vi "Get SMO HELP.vi"(8 "error in (no error)":errorcluster, 10 "Command":string, 11 "Inst.Krohn-Hite-7008 in":refnum<class "Inst.Krohn-Hite-7008.lvclass">) -> (0 "error out":errorcluster, 2 "help cluster":T1, 3 "Inst.Krohn-Hite-7008 out":refnum<class "Inst.Krohn-Hite-7008.lvclass">)   [LabVIEW 2019, in "Inst.Krohn-Hite-7008.lvclass"]
uses:
  Inst.Krohn-Hite-7008.lvclass
  <userlib>/LevyLab/Instrument Framework/subsystems/Help/typedefs/Help--cluster.ctl
  Typedefs/getChannelRequest--Cluster.ctl
  KH7008/typedefs/channel--numeric.ctl
  Typedefs/getAllChannelsResponse--Cluster.ctl
  KH7008/typedefs/allChannelProperties--Array.ctl
  KH7008/typedefs/channelProperties--Cluster.ctl
  KH7008/typedefs/gain--enum.ctl
  KH7008/typedefs/Input--Enum.ctl
  KH7008/typedefs/shunt--enum.ctl
  KH7008/typedefs/couple--Enum.ctl
  KH7008/typedefs/Filter--Enum.ctl
  Typedefs/setChannelRequest--Cluster.ctl
  Typedefs/setAllChannelsRequest--Cluster.ctl
  <userlib>/LevyLab/Instrument Framework/Instrument Types/Amplifier/Instrument.Amplifier.lvclass
  <userlib>/LevyLab/Instrument Framework/subsystems/Help/Help.lvclass
  <userlib>/LevyLab/Instrument Framework/Instrument/Typedefs/Instrument.Commands--Enum.ctl
  <vilib>/PRIrvin/JSON-Schema/JSON-Schema.lvlib
  KH7008/KH7008.lvlib
  <userlib>/LevyLab/Instrument Framework/Instrument/Typedefs/Instrument.IDN--cluster.ctl
  <userlib>/LevyLab/Instrument Framework/Instrument/Instrument.lvclass
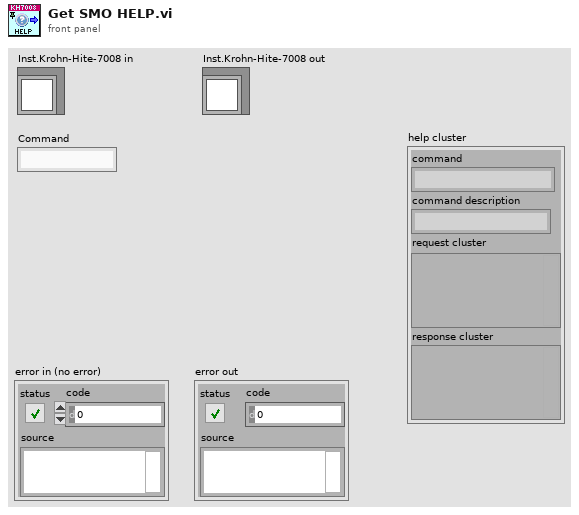
[diagram p1: front panel]
types:
  T1 = typedef "Instrument.lvlib/Help.lvclass/Help--cluster.ctl" = cluster{"command":string, "command description":string, "request cluster":variant, "response cluster":variant}
  T2 = typedef "Inst.Krohn-Hite-7008.lvclass/getAllChannelsResponse--Cluster.ctl" = cluster{"allChannelProperties":T3}
  T3 = typedef "KH7008.lvlib/allChannelProperties--Array.ctl" = T4[]
  T4 = typedef "KH7008.lvlib/channelProperties--Cluster.ctl" = cluster{"channel":T5, "gain":T6, "input":T7, "shunt":T8, "couple":T9, "filter":T10}
  T5 = typedef "KH7008.lvlib/channel--numeric.ctl" = u16
  T6 = typedef "KH7008.lvlib/gain--enum.ctl" = enum16{"1", "10", "100", "1000"}
  T7 = typedef "KH7008.lvlib/Input--Enum.ctl" = enum16{"OFF", "SE+", "SE-", "DIFF"}
  T8 = typedef "KH7008.lvlib/shunt--enum.ctl" = enum16{"Open", "50", "500", "5k", "50k", "10M"}
  T9 = typedef "KH7008.lvlib/couple--Enum.ctl" = enum16{"AC", "DC"}
  T10 = typedef "KH7008.lvlib/Filter--Enum.ctl" = enum16{"OFF", "ON"}
  T11 = typedef "Inst.Krohn-Hite-7008.lvclass/getChannelRequest--Cluster.ctl" = cluster{"channel":T5}
  T12 = typedef "Inst.Krohn-Hite-7008.lvclass/setChannelRequest--Cluster.ctl" = cluster{"channelProperties":T4}
  T13 = typedef "Inst.Krohn-Hite-7008.lvclass/setAllChannelsRequest--Cluster.ctl" = cluster{"allChannelProperties":T3}
  T14 = typedef "Instrument.lvclass/Instrument.Commands--Enum.ctl" = enum16{"ACK", "HELP", "IDN", "getAll", "getAllData"}
  T15 = typedef "Instrument.lvlib/Instrument.lvclass/Instrument.IDN--cluster.ctl" = cluster{"vendor":string, "model":string, "serial":string, "firmware":string}
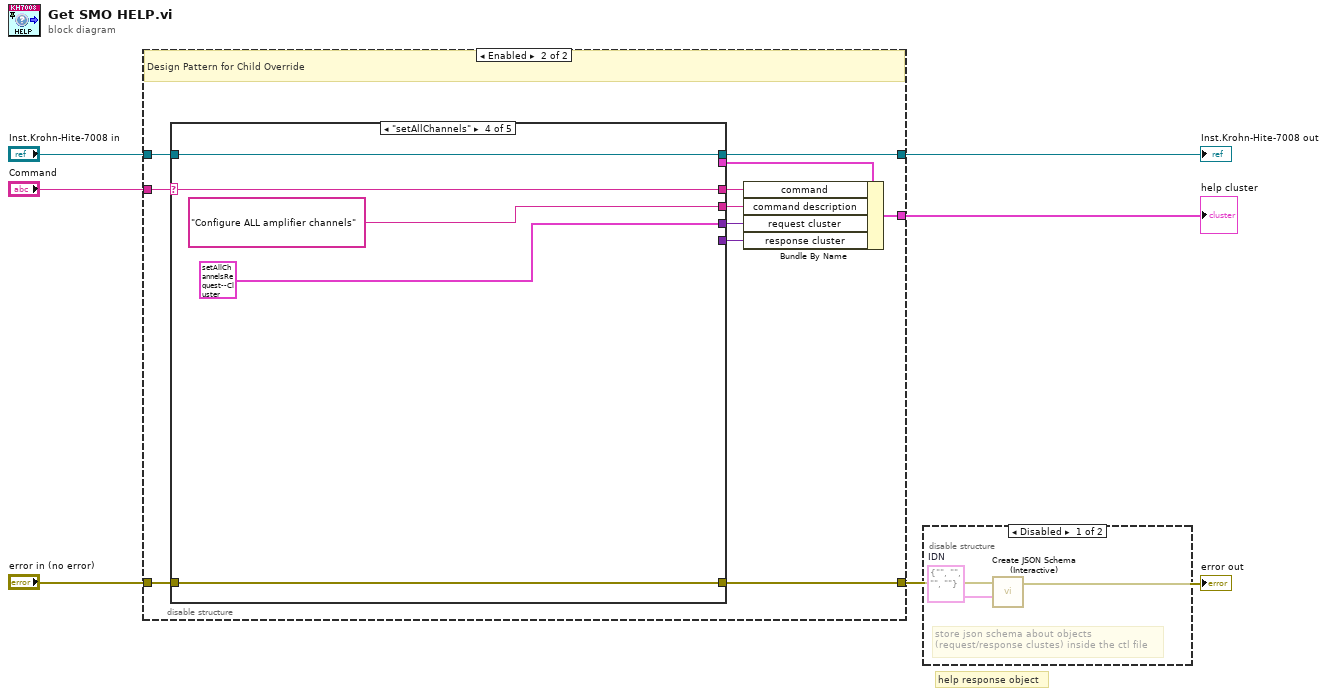
[diagram p0: block diagram]
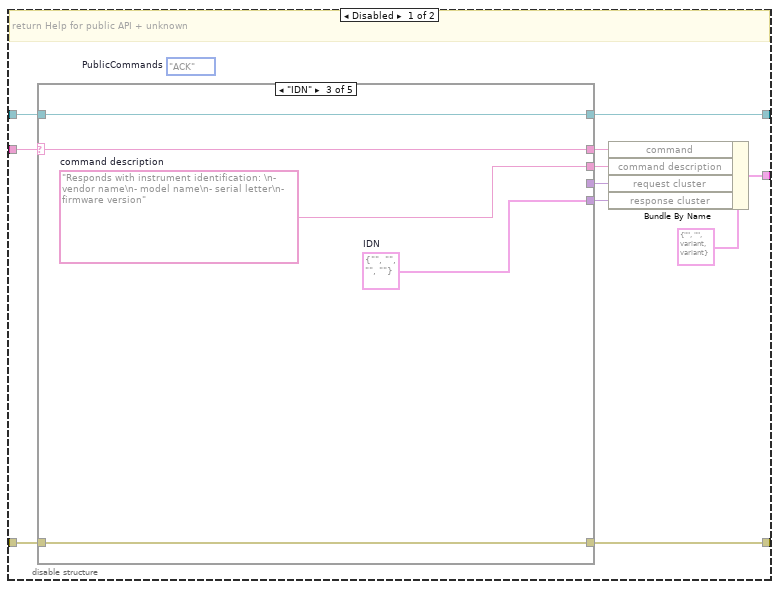
[diagram p2: hidden frame]
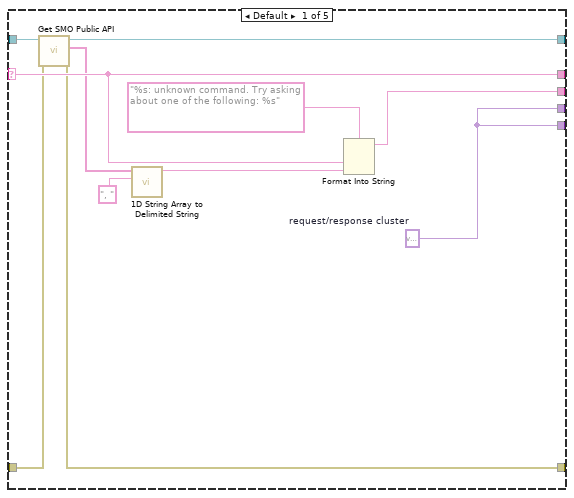
[diagram p3: hidden frame]
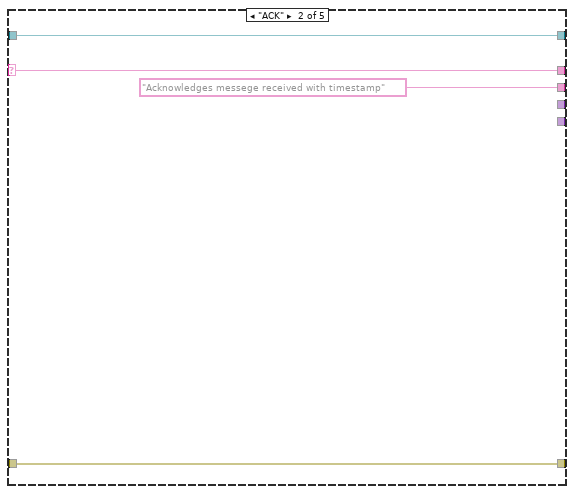
[diagram p4: hidden frame]
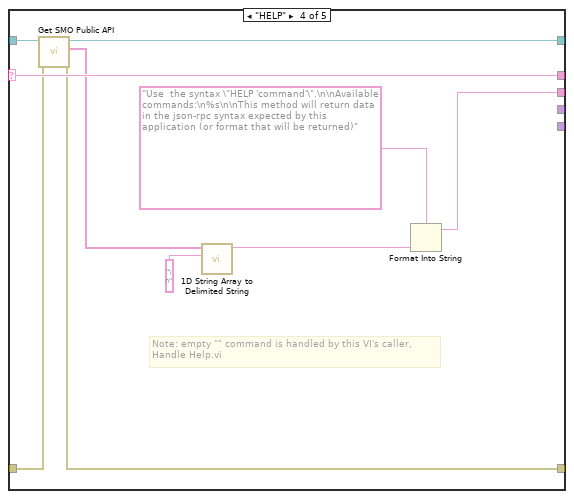
[diagram p5: hidden frame]
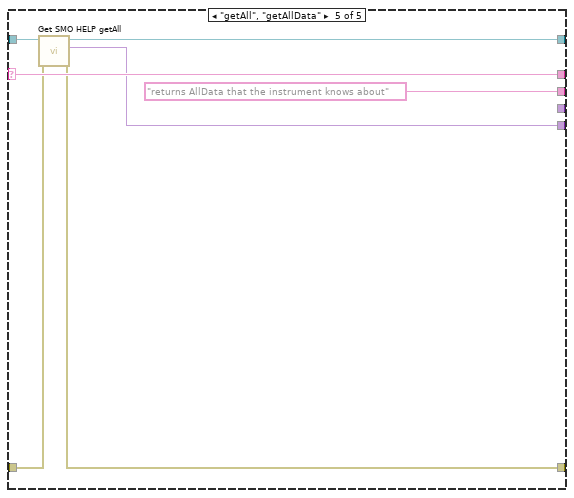
[diagram p6: hidden frame]
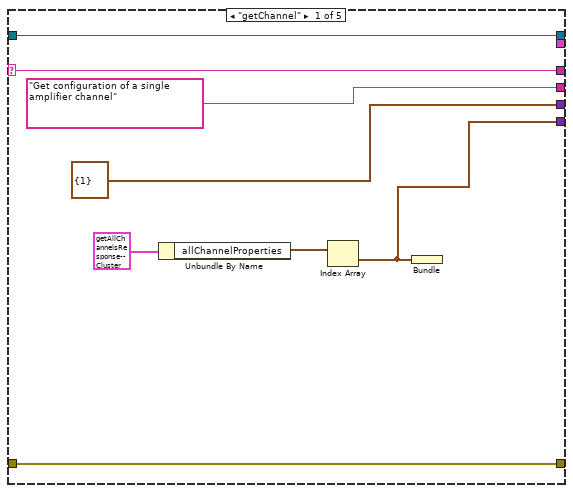
[diagram p7: hidden frame]
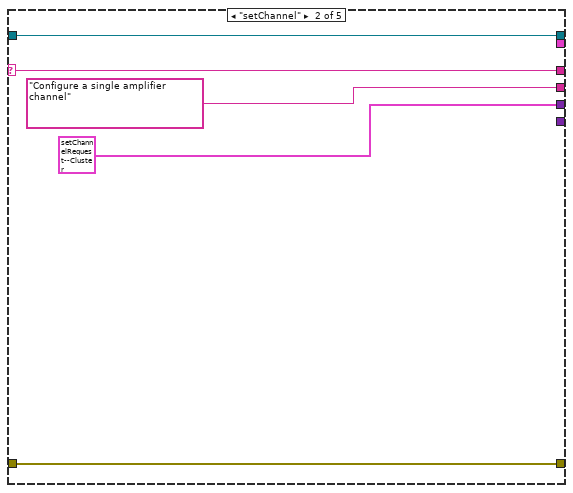
[diagram p8: hidden frame]
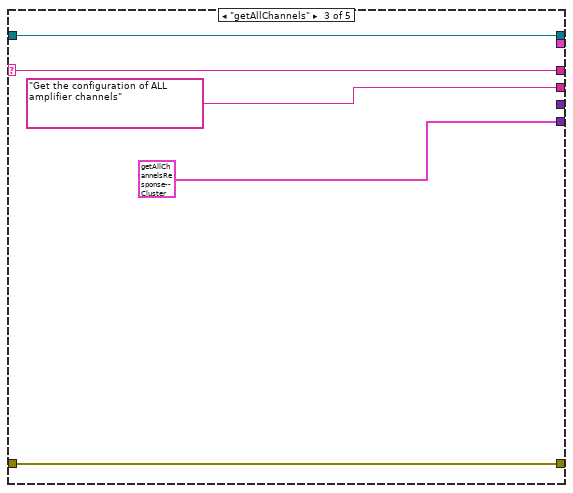
[diagram p9: hidden frame]
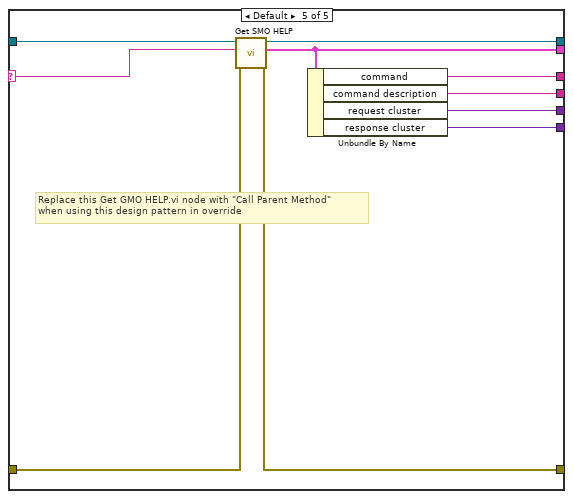
[diagram p10: hidden frame]
diagram:
  # "help response object"
  n1 = disable-structure shown="Enabled" {
    disable-tunnel: [w17 w56] -> w4
    disable-tunnel: "Inst.Krohn-Hite-7008 in" -> [w16 w57]
    disable-tunnel: "error in (no error)" -> [w15 w63]
    disable-tunnel: [w11 w65] -> w6
    disable-tunnel: [w8 w64] -> w5
    disable-tunnel: "Command" -> [w7 w62]
    frame Disabled {
      (unwired) Instrument.Commands--Enum."ACK"  # PublicCommands
      # "return Help for public API + unknown"
      n2 = case shown="\"IDN\"" w7 {
        selector: w7 -> [w24 w30 w36 w44 w53]
        tunnel: w15 -> [w21 w32 w34 w41 w52]
        tunnel: [w22 w32 w34 w42 w51] -> w11
        tunnel: [w26 "Acknowledges messege received with timestamp" w37 w38 "returns AllData that the instrument knows about"] -> w13
        tunnel: [w19 _ _ _ _] -> w12
        tunnel: [w19 _ w33 _ w48] -> w10
        tunnel: [w24 w30 w36 w44 w53] -> w14
        tunnel: w16 -> [w23 w29 w35 w43 w49]
        tunnel: [w20 w29 w35 w40 w50] -> w17
        frame Default {
          w19 = variant  # request/response cluster
          n3 = call-dynamic "Get SMO Public API.vi"("error in (no error)"=w21, "Inst.Krohn-Hite-7008 in"=w23) -> ("error out"=w22:errorcluster, "Commands"=w18:string[], "Inst.Krohn-Hite-7008 out"=w20:refnum<class "Inst.Krohn-Hite-7008.lvclass">)  [unwired: 7 in]
          n4 = call <vilib>:"1D String Array to Delimited String.vi"("delimiter"=", ", "string array"=w18) -> ("delimited string"=w27:string)  [unwired: 9 in]
          n5 = Format Into String(format string="%s: unknown command. Try asking about one of the following: %s", w24, w27) -> (resulting string=w26:string)  [unwired: 2 in, 1 out]
        }
        frame "ACK" {
        }
        frame "IDN" {
          w33 = T15 {"vendor"="", "model"="", "serial"="", "firmware"=""}  # IDN
          w37 = "Responds with instrument identification: \n- vendor name\n- model name\n- serial letter\n- firmware version"  # command description
        }
        frame "HELP" {
          # "Note: empty \"\" command is handled by this VI's caller,\nHandle Help.vi"
          n6 = call-dynamic "Get SMO Public API.vi"("error in (no error)"=w41, "Inst.Krohn-Hite-7008 in"=w43) -> ("error out"=w42:errorcluster, "Commands"=w39:string[], "Inst.Krohn-Hite-7008 out"=w40:refnum<class "Inst.Krohn-Hite-7008.lvclass">)  [unwired: 7 in]
          n7 = call <vilib>:"1D String Array to Delimited String.vi"("delimiter"="\n", "string array"=w39) -> ("delimited string"=w47:string)  [unwired: 9 in]
          n8 = Format Into String(format string="Use  the syntax \"HELP 'command'\".\n\nAvailable commands:\n%s\n\nThis method will return data in the json-rpc syntax expected by this application (or format that will be returned)", w47) -> (resulting string=w38:string)  [unwired: 2 in, 1 out]
        }
        frame "getAll", "getAllData" {
          n9 = call-dynamic "Get SMO HELP getAll.vi"("error in (no error)"=w52, "Inst.Krohn-Hite-7008 in"=w49) -> ("error out"=w51:errorcluster, "response cluster"=w48:variant, "Inst.Krohn-Hite-7008 out"=w50:refnum<class "Inst.Krohn-Hite-7008.lvclass">)  [unwired: 7 in]
        }
      }
      n10 = Bundle By Name(cluster=T1 {"command"="", "command description"="", "request cluster"=variant, "response cluster"=variant} ("Help"), "command"=w14, "command description"=w13, "request cluster"=w12, "response cluster"=w10) -> (w8:T1)
    }
    frame Enabled {
      # "Design Pattern for Child Override"
      n11 = case shown="\"setAllChannels\"" w62 {
        selector: w62 -> [w73 w78 w83 w88 w97]
        tunnel: [w73 w78 w83 w88 w92] -> w61
        tunnel: w63 -> [w72 w77 w82 w87 w90]
        tunnel: [w72 w77 w82 w87 w89] -> w65
        tunnel: ["Get configuration of a single amplifier channel" "Configure a single amplifier channel" "Get the configuration of ALL amplifier channels" "Configure ALL amplifier channels" w93] -> w60
        tunnel: [T11 {"channel"=1} ("getChannelRequest") T12 {"channelProperties"={"channel"=1, "gain"=enum."10", "input"=enum."OFF", "shunt"=enum."10M", "couple"=enum."AC", "filter"=enum."OFF"}} ("setChannelRequest") _ T13 {"allChannelProperties"=[{"channel"=1, "gain"=enum."10", "input"=enum."OFF", "shunt"=enum."10M", "couple"=enum."AC", "filter"=enum."OFF"}, {"channel"=2, "gain"=enum."10", "input"=enum."OFF", "shunt"=enum."10M", "couple"=enum."AC", "filter"=enum."OFF"}, {"channel"=3, "gain"=enum."10", "input"=enum."OFF", "shunt"=enum."10M", "couple"=enum."AC", "filter"=enum."OFF"}, {"channel"=4, "gain"=enum."10", "input"=enum."OFF", "shunt"=enum."10M", "couple"=enum."AC", "filter"=enum."OFF"}, {"channel"=5, "gain"=enum."10", "input"=enum."OFF", "shunt"=enum."10M", "couple"=enum."AC", "filter"=enum."OFF"}, {"channel"=6, "gain"=enum."10", "input"=enum."OFF", "shunt"=enum."10M", "couple"=enum."AC", "filter"=enum."OFF"}, {"channel"=7, "gain"=enum."10", "input"=enum."OFF", "shunt"=enum."10M", "couple"=enum."AC", "filter"=enum."OFF"}, {"channel"=7, "gain"=enum."10", "input"=enum."OFF", "shunt"=enum."10M", "couple"=enum."AC", "filter"=enum."OFF"}]} ("setAllChannelsRequest") w94] -> w59
        tunnel: [w67 _ T2 {"allChannelProperties"=[{"channel"=1, "gain"=enum."10", "input"=enum."OFF", "shunt"=enum."10M", "couple"=enum."AC", "filter"=enum."OFF"}, {"channel"=2, "gain"=enum."10", "input"=enum."OFF", "shunt"=enum."10M", "couple"=enum."AC", "filter"=enum."OFF"}, {"channel"=3, "gain"=enum."10", "input"=enum."OFF", "shunt"=enum."10M", "couple"=enum."AC", "filter"=enum."OFF"}, {"channel"=4, "gain"=enum."10", "input"=enum."OFF", "shunt"=enum."10M", "couple"=enum."AC", "filter"=enum."OFF"}, {"channel"=5, "gain"=enum."10", "input"=enum."OFF", "shunt"=enum."10M", "couple"=enum."AC", "filter"=enum."OFF"}, {"channel"=6, "gain"=enum."10", "input"=enum."OFF", "shunt"=enum."10M", "couple"=enum."AC", "filter"=enum."OFF"}, {"channel"=7, "gain"=enum."10", "input"=enum."OFF", "shunt"=enum."10M", "couple"=enum."AC", "filter"=enum."OFF"}, {"channel"=7, "gain"=enum."10", "input"=enum."OFF", "shunt"=enum."10M", "couple"=enum."AC", "filter"=enum."OFF"}]} ("getAllChannelsResponse") _ w95] -> w58
        tunnel: w57 -> [w70 w75 w80 w85 w98]
        tunnel: [w70 w75 w80 w85 w96] -> w56
        tunnel: [_ _ _ _ w91] -> w55
        frame "getChannel" {
          n12 = Unbundle By Name(T2 {"allChannelProperties"=[{"channel"=1, "gain"=enum."10", "input"=enum."OFF", "shunt"=enum."10M", "couple"=enum."AC", "filter"=enum."OFF"}, {"channel"=2, "gain"=enum."10", "input"=enum."OFF", "shunt"=enum."10M", "couple"=enum."AC", "filter"=enum."OFF"}, {"channel"=3, "gain"=enum."10", "input"=enum."OFF", "shunt"=enum."10M", "couple"=enum."AC", "filter"=enum."OFF"}, {"channel"=4, "gain"=enum."10", "input"=enum."OFF", "shunt"=enum."10M", "couple"=enum."AC", "filter"=enum."OFF"}, {"channel"=5, "gain"=enum."10", "input"=enum."OFF", "shunt"=enum."10M", "couple"=enum."AC", "filter"=enum."OFF"}, {"channel"=6, "gain"=enum."10", "input"=enum."OFF", "shunt"=enum."10M", "couple"=enum."AC", "filter"=enum."OFF"}, {"channel"=7, "gain"=enum."10", "input"=enum."OFF", "shunt"=enum."10M", "couple"=enum."AC", "filter"=enum."OFF"}, {"channel"=7, "gain"=enum."10", "input"=enum."OFF", "shunt"=enum."10M", "couple"=enum."AC", "filter"=enum."OFF"}]} ("getAllChannelsResponse")) -> ("allChannelProperties"=w68:T3)
          n13 = Index Array(array=w68) -> (element=w67:T4)  [unwired: 1 in]
          n14 = Bundle("channelProperties"=w67) -> ()  [unwired: 1 in, 1 out]
        }
        frame "setChannel" {
        }
        frame "getAllChannels" {
        }
        frame "setAllChannels" {
        }
        frame Default {
          # "Replace this Get GMO HELP.vi node with \"Call Parent Method\"\nwhen using this design pattern in override"
          n15 = call-parent "Get SMO HELP.vi"("error in (no error)"=w90, "Command"=w97, "Instrument.Amplifier in"=w98) -> ("error out"=w89:errorcluster, "help cluster"=w91:T1, "Instrument.Amplifier out"=w96:refnum<class "Inst.Krohn-Hite-7008.lvclass">)  [unwired: 6 in]
          n16 = Unbundle By Name(w91) -> ("command"=w92:string, "command description"=w93:string, "request cluster"=w94:variant, "response cluster"=w95:variant)
        }
      }
      n17 = Bundle By Name(cluster=w55, "command"=w61, "command description"=w60, "request cluster"=w59, "response cluster"=w58) -> (w64:T1)
    }
  }
  "Inst.Krohn-Hite-7008 out" <- w4
  "help cluster" <- w5
  "error out" <- w6
  n18 = disable-structure shown="Disabled" {
    frame Disabled {
      w99 = T15 {"vendor"="", "model"="", "serial"="", "firmware"=""}  # IDN
      # "store json schema about objects\n(request/response clustes) inside the ctl file"
      n19 = call <vilib>:"Create JSON Schema (Interactive).vi"("LV Object"=w99) -> ()  [unwired: 9 in, 2 out]
    }
    frame Enabled {
    }
  }
